vi "Initialize Acquisition.vi"(8 "error in":errorcluster, 11 "DAQmxChannel":T1) -> (0 "error out":errorcluster, 3 "task out":refnum<k21>)   [LabVIEW 2018]
doc: "Konfiguruje kana³ pomiarowy karty DAQ do pomiaru napiêcia i wyzwala start akwizycji."
uses:
  controls/Daqtypedef.ctl
  <vilib>/DAQmx/create/channels.llb/DAQmx Create Channel (AI-Voltage-Basic).vi
  <vilib>/DAQmx/configure/timing.llb/DAQmx Timing (Sample Clock).vi
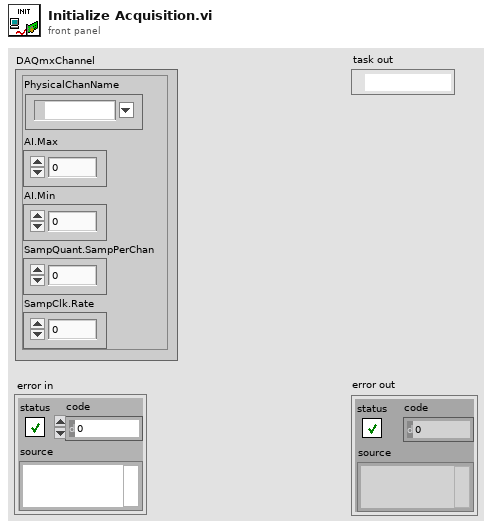
[diagram p1: front panel]
types:
  T1 = typedef "Daqtypedef.ctl" = cluster{"PhysicalChanName":tag, "AI.Max":dbl, "AI.Min":dbl, "SampQuant.SampPerChan":i32, "SampClk.Rate":dbl}
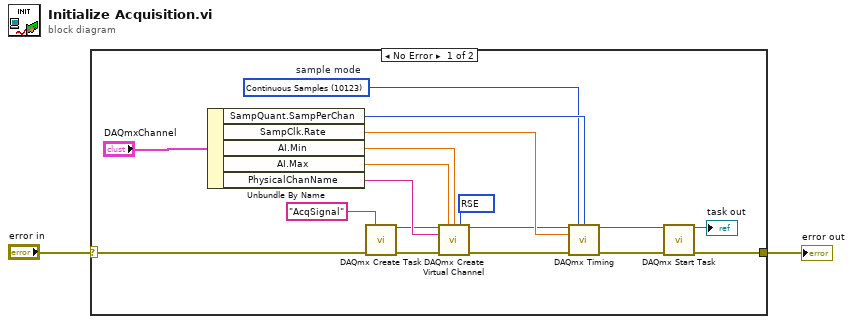
[diagram p0: block diagram]
diagram:
  n1 = case shown="No Error" "error in" {
    selector: "error in" -> [w10 w21]
    tunnel: [w9 w21] -> w2
    frame No Error {
      w3 = 10083 items=["Default"=-1, "RSE"=10083, "NRSE"=10078, "Differential"=10106, "Pseudodifferential"=12529] ("input terminal configuration")
      w14 = 10123 items=["Finite Samples"=10178, "Continuous Samples"=10123, "Hardware Timed Single Point"=12522]  # sample mode
      n2 = Unbundle By Name("DAQmxChannel") -> ("SampQuant.SampPerChan"=w16:i32, "SampClk.Rate"=w15:dbl, "AI.Min"=w19:dbl, "AI.Max"=w18:dbl, "PhysicalChanName"=w17:tag)
      n3 = call <vilib>:"DAQmx Create Task.vi"("new task name"="AcqSignal", "error in"=w10) -> ("task out"=w5:refnum<k21>, "error out"=w6:errorcluster)  [unwired: 12 in]
      n4 = call-poly <vilib>:"DAQmx Create Virtual Channel.vi"("task in"=w5, "maximum value"=w18, "minimum value"=w19, "input terminal configuration"=w3, "physical channels"=w17, "error in"=w6) -> ("task out"=w12:refnum<k21>, "error out"=w13:errorcluster)  [unwired: 8 in]
      n5 = call-poly <vilib>:"DAQmx Timing.vi"("task/channels in"=w12, "sample mode"=w14, "samples per channel"=w16, "rate"=w15, "error in"=w13) -> ("task out"=w8:refnum<k21>, "error out"=w11:errorcluster)  [unwired: 9 in]
      n6 = call <vilib>:"DAQmx Start Task.vi"("task/channels in"=w8, "error in"=w11) -> ("task out"=→"task out":refnum<k21>, "error out"=w9:errorcluster)  [unwired: 12 in]
    }
    frame Error {
    }
  }
  "error out" <- w2
